vi "SV TDMS Write X Properties.vi"(0 "tdms file in":refnum<k34>, 1 "X-axis label":string, 2 "X-unit string":string, 5 "group name":string, 7 "channel name":string, 11 "error in":errorcluster) -> (4 "tdms file out":refnum<k34>, 6 "group name":string, 8 "channel name":string, 15 "error out":errorcluster)   [LabVIEW 2017]
uses:
  <vilib>/addons/_NISVFA/_Shared subVIs/Controls/NI Channel Properties.ctl
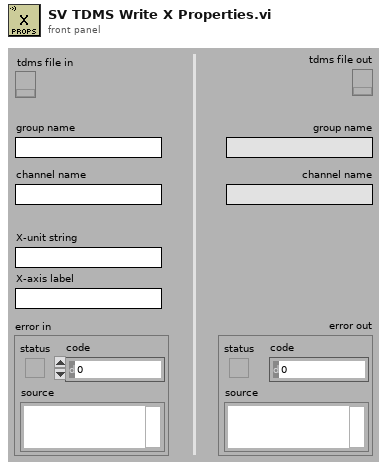
[diagram p1: front panel]
types:
  T1 = typedef "NI Channel Properties.ctl" = u16
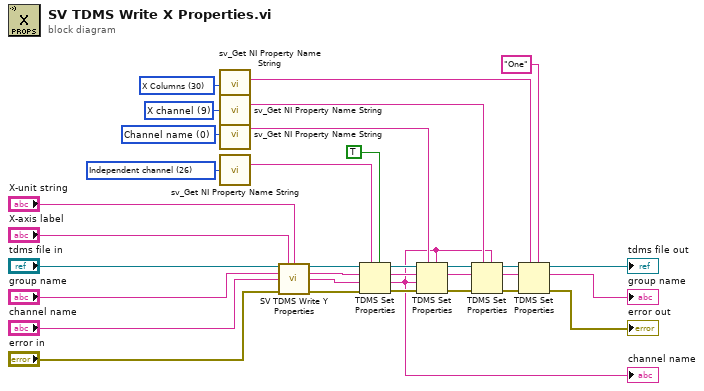
[diagram p0: block diagram]
diagram:
  w23 = T1 30 items=["Channel name", "Channel description", "Axis label", "Unit string", "Waveform X-axis label", "Waveform X-axis unit string", "x0", "dx", "Number of samples", "X channel", "Filter settled", "dB reference", "Window", "Window parameter", "Window size", "FFT size", "Peak units", "Spectrum type", "Magnitude scale", "Spectral density", "Sensor sensitivity (mV/EU)", "X-axis dimension", "LabVIEW datatype", "Function type", "Function subtype", "X values", "Independent channel", "Column index", "Collection name", "Collection ID", "X Columns"] ("property")
  w13 = T1 0 items=["Channel name", "Channel description", "Axis label", "Unit string", "Waveform X-axis label", "Waveform X-axis unit string", "x0", "dx", "Number of samples", "X channel", "Filter settled", "dB reference", "Window", "Window parameter", "Window size", "FFT size", "Peak units", "Spectrum type", "Magnitude scale", "Spectral density", "Sensor sensitivity (mV/EU)", "X-axis dimension", "LabVIEW datatype", "Function type", "Function subtype", "X values", "Independent channel"] ("property")
  w22 = T1 26 items=["Channel name", "Channel description", "Y-axis label", "Y-axis unit string", "X-axis label", "X-axis unit string", "x0", "dx", "Number of samples", "X channel", "Filter settled", "dB reference", "Window", "Window parameter", "Window size", "FFT size", "Peak units", "Spectrum type", "Magnitude scale", "Spectral density", "Sensor sensitivity (mV/EU)", "X-axis dimension", "LabVIEW datatype", "Function type", "Function subtype", "X values", "Independent channel"] ("property")
  w33 = T1 9 items=["Channel name", "Channel description", "Y-axis label", "Y-axis unit string", "X-axis label", "X-axis unit string", "x0", "dx", "Number of samples", "X channel", "Filter settled", "dB reference", "Window", "Window parameter", "Window size", "FFT size", "Peak units", "Spectrum type", "Magnitude scale", "Spectral density", "Sensor sensitivity (mV/EU)", "X-axis dimension", "LabVIEW datatype", "Function type", "Function subtype", "X-values"] ("property")
  n1 = call <vilib>:"sv_Get NI Property Name String.vi"("property"=w23) -> ("TDMS property name"=w25:string)  [unwired: 13 in, 1 out]
  n2 = call <vilib>:"sv_Get NI Property Name String.vi"("property"=w33) -> ("TDMS property name"=w32:string)  [unwired: 13 in, 1 out]
  n3 = call <vilib>:"sv_Get NI Property Name String.vi"("property"=w13) -> ("TDMS property name"=w12:string)  [unwired: 13 in, 1 out]
  n4 = call <vilib>:"sv_Get NI Property Name String.vi"("property"=w22) -> ("TDMS property name"=w21:string)  [unwired: 13 in, 1 out]
  n5 = call <vilib>:"SV TDMS Write Y Properties.vi"("tdms file"="tdms file in", "y-axis label"="X-axis label", "y-unit string"="X-unit string", "group name"="group name", "channel name"="channel name", "error in (no error)"="error in") -> ("tdms file out"=w4:refnum<k34>, "group name"=w3:string, "channel name"=w2:string, "error out"=w1:errorcluster)  [unwired: 6 in]
  n6 = TDMS Set Properties(5:TRUE, 7:w21, 8:w1, 9:w2, 10:w3, 11:w4) -> (0:w14:errorcluster, 1:w11:string, 2:w18:string, 3:w19:refnum<k34>)
  "channel name" <- w11
  n7 = TDMS Set Properties(5:w11, 7:w12, 8:w14, 9:w11, 10:w18, 11:w19) -> (0:w15:errorcluster, 2:w16:string, 3:w17:refnum<k34>)  [unwired: 1 out]
  n8 = TDMS Set Properties(5:w11, 7:w32, 8:w15, 10:w16, 11:w17) -> (0:w31:errorcluster, 2:w30:string, 3:w29:refnum<k34>)  [unwired: 1 in, 1 out]
  n9 = TDMS Set Properties(5:"One" ("TDMS property name"), 7:w25, 8:w31, 10:w30, 11:w29) -> (0:→"error out":errorcluster, 2:→"group name":string, 3:→"tdms file out":refnum<k34>)  [unwired: 1 in, 1 out]
